vi "Main.vi"() -> ()   [LabVIEW 2017]
doc: "Use this template to build a user interface event handler design pattern. Use this pattern for dialog boxes and other user interfaces. You also can create and execute user-defined events that the VI can handle the same way as user interface events."
uses:
  <vilib>/Utility/NIReport.llb/HTML Report Image Alignment.ctl
  <vilib>/Utility/NIReport.llb/image depth.ctl
  <vilib>/addons/database/Connection.llb/DB Tools Open Connec (Path).vi
  <userlib>/_OpenG.lib/file/file.llb/File Exists - Scalar__ogtk.vi
  <vilib>/addons/database/Auxilliary.llb/DB Tools Format Datetime String (Time Stamp).vi
  GLOBAL/auto.vi
  <vilib>/Utility/NIReport.llb/Append Report Text (str wrap).vi
  <vilib>/Utility/NIReport.llb/NI_report.lvclass
  <vilib>/addons/database/NI_Database_API.lvlib
  <vilib>/Utility/NIReport.llb/NI_ReportGenerationCore.lvlib
  <vilib>/Utility/NIReport.llb/Excel/NI_Excel.lvclass
panel:
  out "columns":string[](array[string])
  in  "MAX MIN VALUES":enum32{"ACTUAL", "SET"}(tab)
  out "TEMP":cluster{"MIN":dbl, "MAX":dbl, "ACTUAL":dbl}
  out "FLOW":cluster{"MIN":dbl, "MAX":dbl, "ACTUAL":dbl}
  out "BMP":cluster{"ACTUAL":dbl}
  out "Pressure":cluster{"MIN":dbl, "MAX":dbl, "ACTUAL":dbl}
  out "TEMP SET":cluster{"MIN":dbl, "MAX":dbl, "THRESHOLD":dbl}
  out "FLOW SET":cluster{"MIN":dbl, "MAX":dbl, "THRESHOLD":dbl}
  out "BMP SET":cluster{"MIN":dbl, "MAX":dbl, "THRESHOLD":dbl}
  out "Pressure SET":cluster{"MIN":dbl, "MAX":dbl, "THRESHOLD":dbl}
  out "Loading....":u8(slide) scale=0.0..100.0
  out "BMP":bool
  out "Temp":bool
  out "Flow":bool
  out "Pressure":bool
  in  "Report":bool
  out "DESCRIPTION":string
  out "resulting string":path
  in  "import state 3":bool
  out "User Name":string
  out "Min Peak/Min":dbl
  out "Status bar":string
  in  "import state 2":bool
  out "SELECTED RECIPE":string
  out "BARCODE_FOUND":bool
  out "DB CONN":bool
  in  "Graph":bool
  out "table":string[][](table)
  out "GRAPH":cluster{timestamp[], ext[]}[](graph)
  out "TEST RESULT":bool
  in  "BARCODE":string
  out "SELECTED FILE PATH":path
  in  "Import File":bool
  in  "SELECT MEASURED FILE":i32(listbox)
  out "error out":errorcluster
  in  "File Name":string
  in  "Report Files Folder":path
  in  "Convert":bool
  in  "BROWSE FILE FOLDER":path=path "D:/ON FLOOR/Grandiose Automation/Ref Data/Test reading - 141221"
  in  "stop":bool
  # "Main"
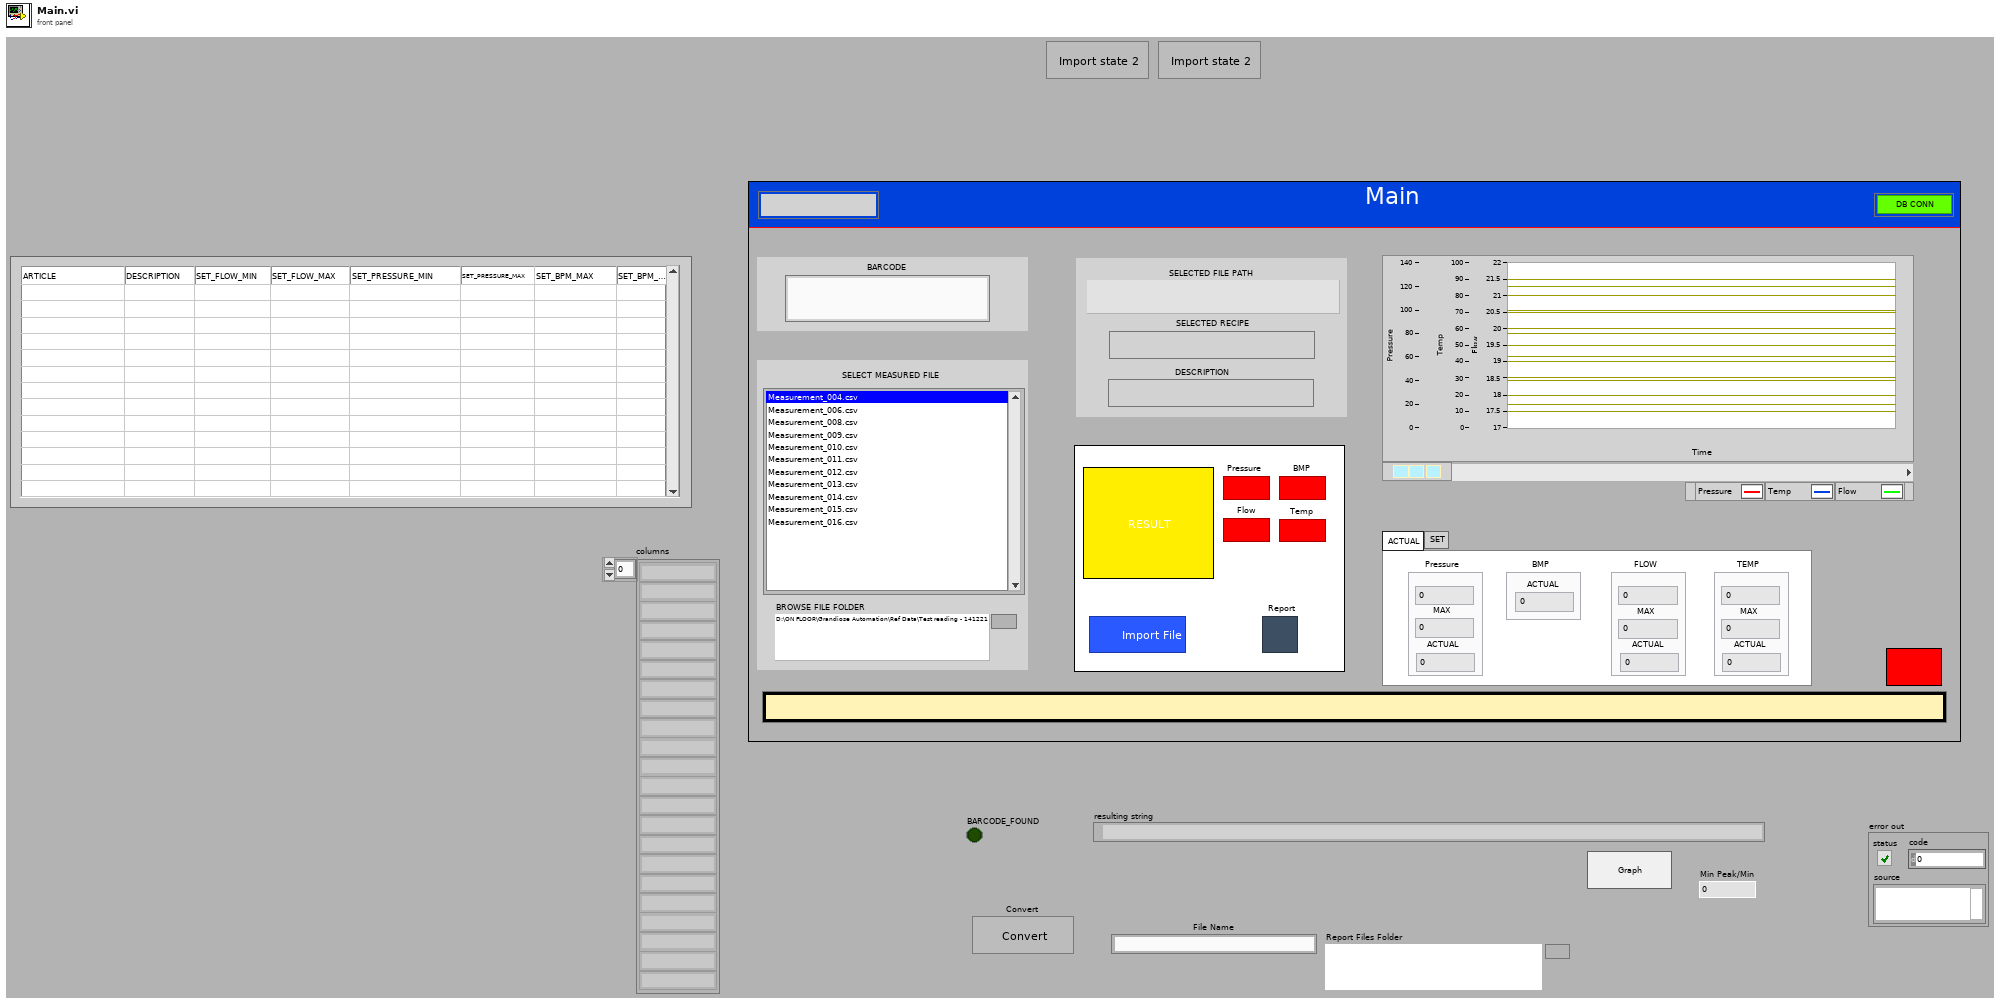
[diagram p1: front panel]
types:
  T1 = cluster{"Files":string[], "Browse File":path, "TIMEOUT":i32, "GRAPH":cluster{timestamp[], ext[]}[], "Pressure":cluster{"chl1 MIN":dbl, "chl1 MAX":dbl, "chl1 thrshold":dbl}, "Flow":cluster{"chl2 MIN":dbl, "chl2 MAX":dbl, "chl2 thrshold":dbl}, "Temp":cluster{"chl3 MIN":dbl, "chl3 MAX":dbl, "chl3 thrshold":dbl}, "Report File":path, "Data_to_report":cluster{"date/time string":string, "User Name":string, "BARCODE":string, "SELECTED RECIPE":string, "Rst":string, "Error Code":string, "RESULT ARRAY":string[]}, "BMP":cluster{"chl3 MIN":dbl, "chl3 MAX":dbl, "chl3 thrshold":dbl}}
  T2 = typedef "NI_Database_API.lvlib/Conn ObjectReference.ctl" = refnum<k1>
  T3 = enum32{"Invalid", "Standard", "Closed", "Hidden", "Minimized", "Maximized"}
  T4 = cluster{"position (Excel)":cluster{"row":i32, "column":i32}, "name (Excel)":string, "bookmark (Word)":string}[]
  T5 = cluster{"position (Excel)":cluster{"row":i32, "column":i32}, "name (Excel)":string, "bookmark (Word)":string}
  T6 = typedef "NI_ReportGenerationCore.lvlib/HTML Report Image Alignment.ctl" = enum16{"(default)", "LEFT", "RIGHT", "TOP", "TEXTTOP", "MIDDLE", "ABSMIDDLE", "BASELINE", "BOTTOM", "ABSBOTTOM"}
  T7 = enum16{"Standard Report", "HTML", "Word", "Excel"}
  T8 = enum16{"maximized", "minimized", "normal", "no change"}
  T9 = cluster{"Pressure":cluster{"chl1 MIN":dbl, "chl1 MAX":dbl, "chl1 thrshold":dbl}, "Flow":cluster{"chl2 MIN":dbl, "chl2 MAX":dbl, "chl2 thrshold":dbl}, "Temp":cluster{"chl3 MIN":dbl, "chl3 MAX":dbl, "chl3 thrshold":dbl}, "BMP":cluster{"chl3 MIN":dbl, "chl3 MAX":dbl, "chl3 thrshold":dbl}}
  T10 = cluster{"chl1 MIN":dbl, "chl1 MAX":dbl, "chl1 thrshold":dbl}
  T11 = cluster{"chl2 MIN":dbl, "chl2 MAX":dbl, "chl2 thrshold":dbl}
  T12 = cluster{"chl3 MIN":dbl, "chl3 MAX":dbl, "chl3 thrshold":dbl}
  T13 = cluster{"date/time string":string, "User Name":string, "BARCODE":string, "SELECTED RECIPE":string, "Rst":string, "Error Code 2":string}
  T14 = cluster{"date/time string":string, "User Name":string, "BARCODE":string, "SELECTED RECIPE":string, "Rst":string, "Error Code 2":string, "element":string, "element":string, "element":string, "element":string, "element":string, "element":string, "element":string, "element":string, "element":string, "element":string, "element":string}
  T15 = cluster{"date/time string":string, "User Name":string, "BARCODE":string, "SELECTED RECIPE":string, "Rst":string, "Error Code 2":string, "RESULT ARRAY":string[]}
  T16 = typedef "NI_ReportGenerationCore.lvlib/image depth.ctl" = u16
  T17 = enum32{"invalid app kind", "Development System", "Run Time System", "Student Edition", "Embedded LabVIEW", "Evaluation", "Custom"}
  T18 = cluster{"date/time string":string, "User Name":string, "BARCODE":string, "SELECTED RECIPE":string, "Rst":string, "Error Code":string, "RESULT ARRAY":string[]}
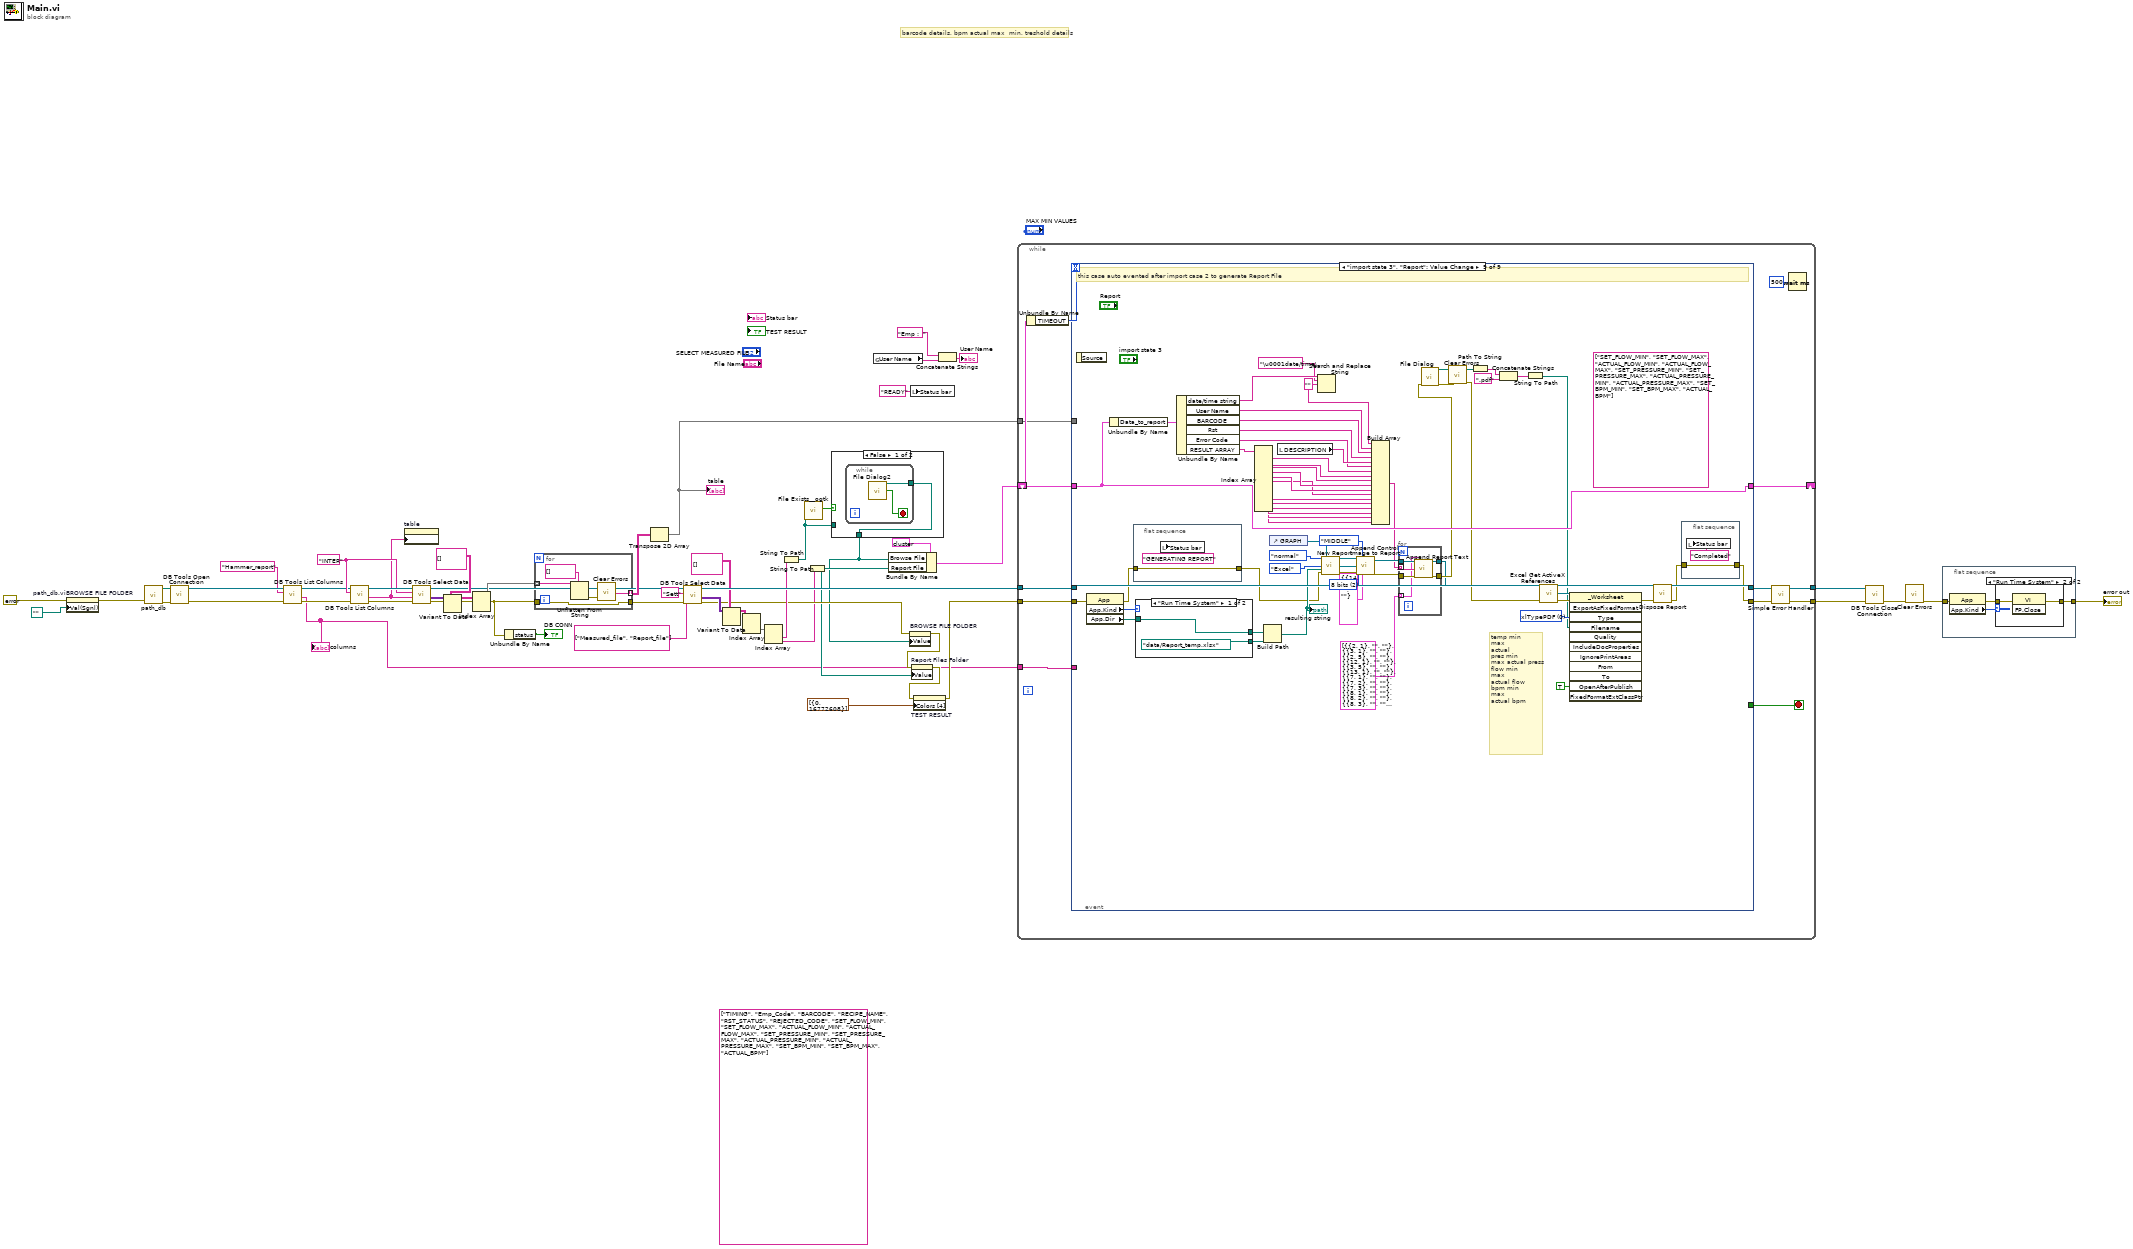
[diagram p0: block diagram]
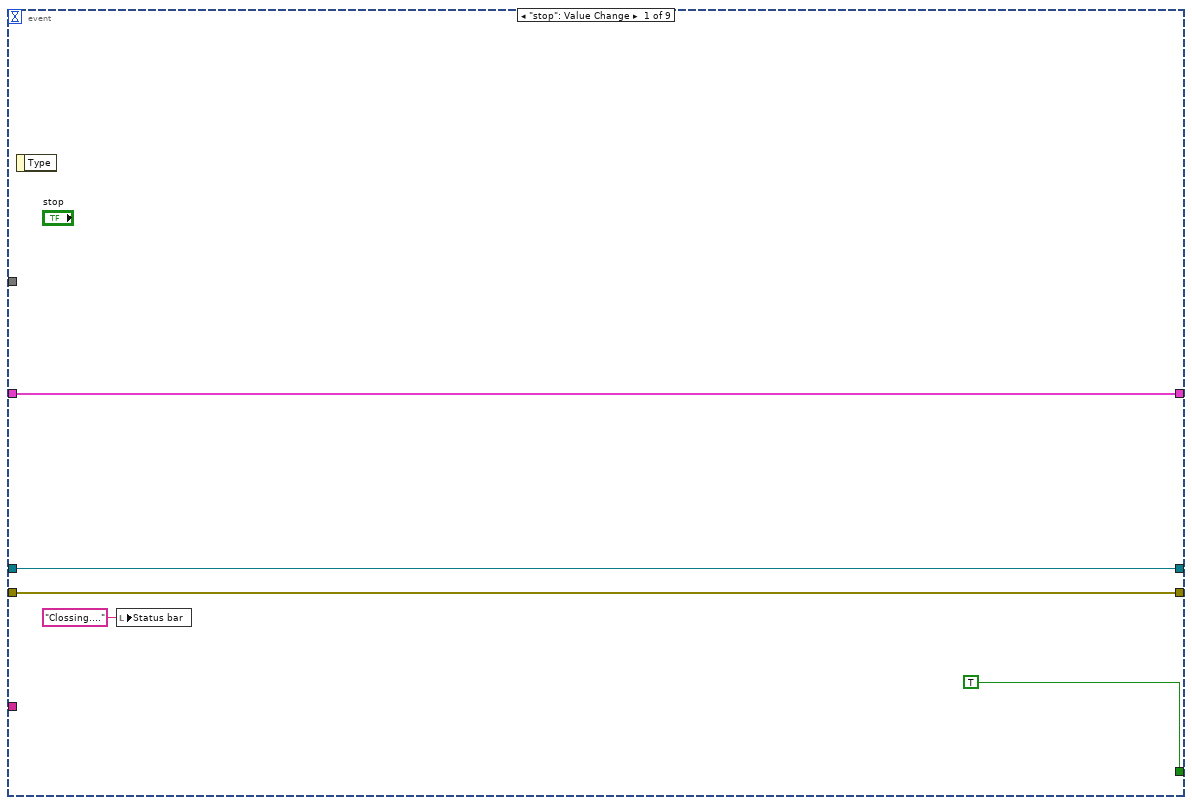
[diagram p4: hidden frame]
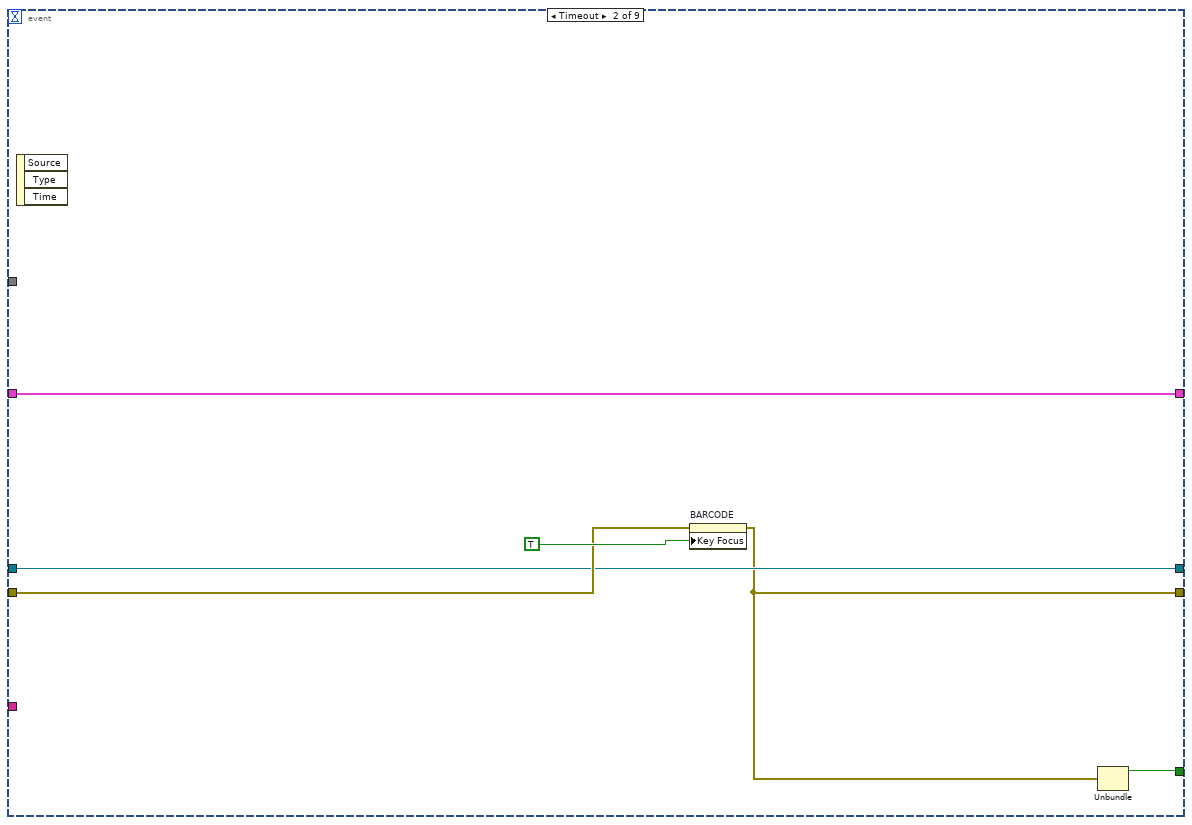
[diagram p5: hidden frame]
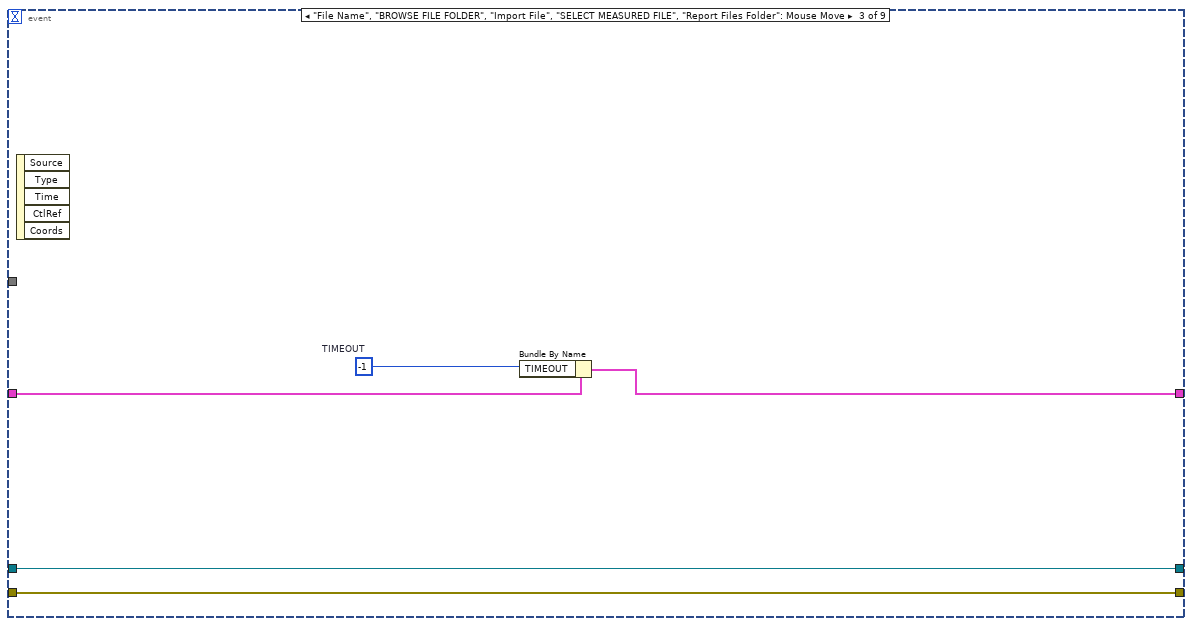
[diagram p6: hidden frame]
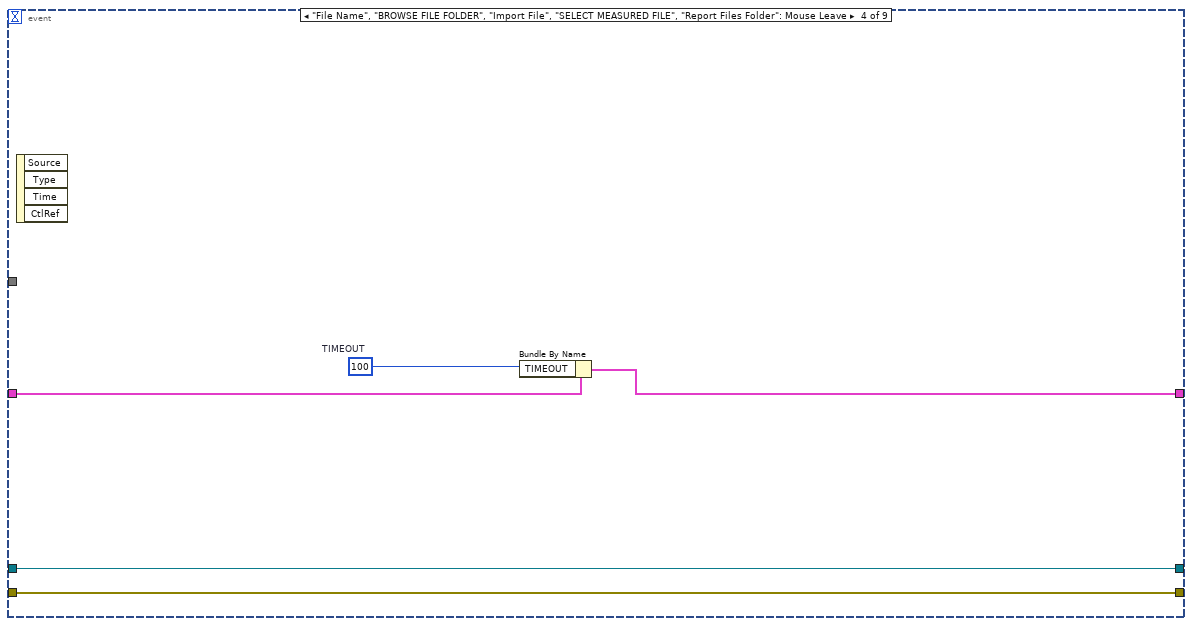
[diagram p7: hidden frame]
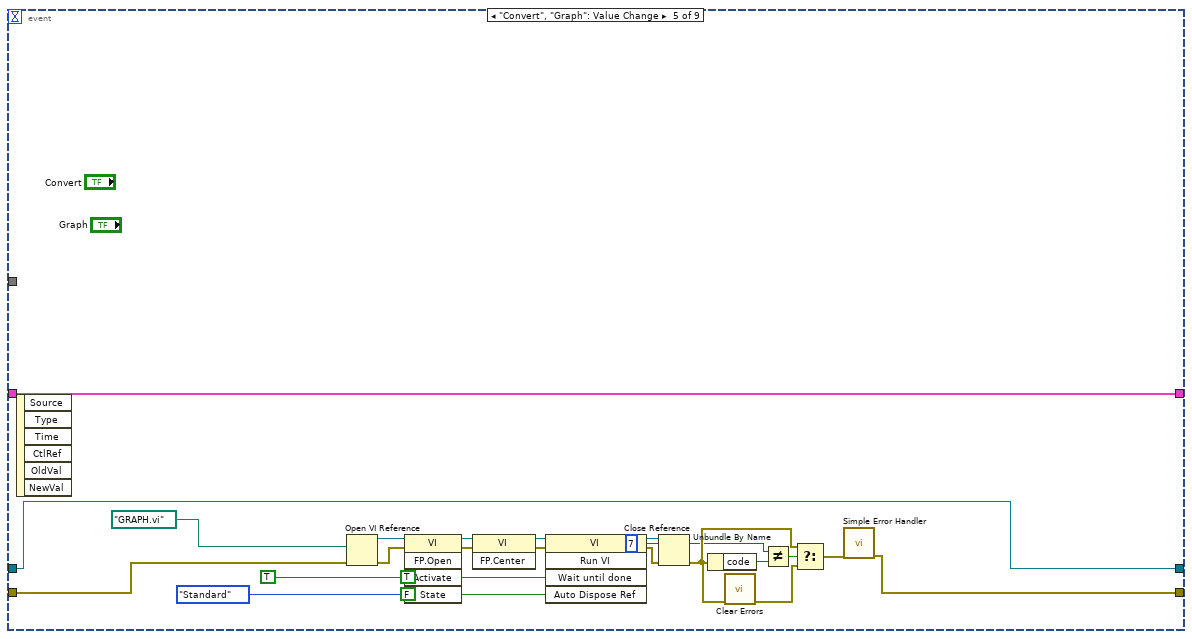
[diagram p8: hidden frame]
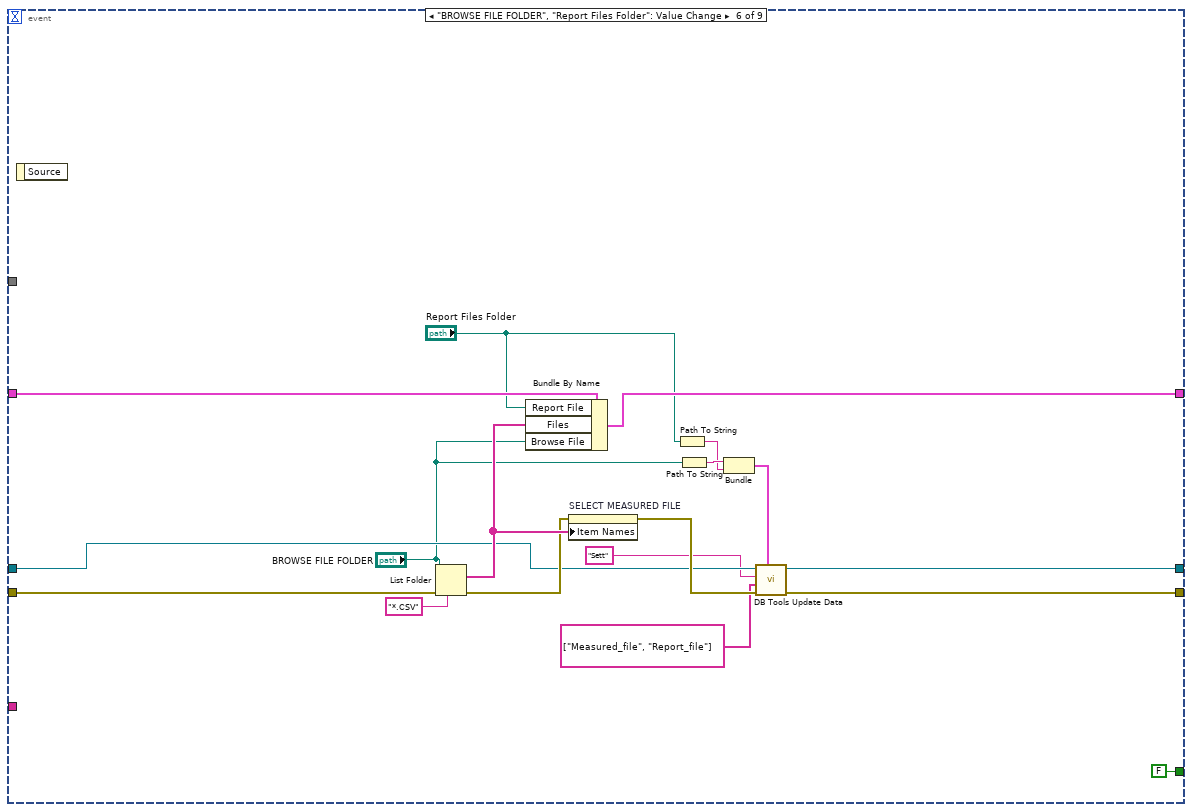
[diagram p9: hidden frame]
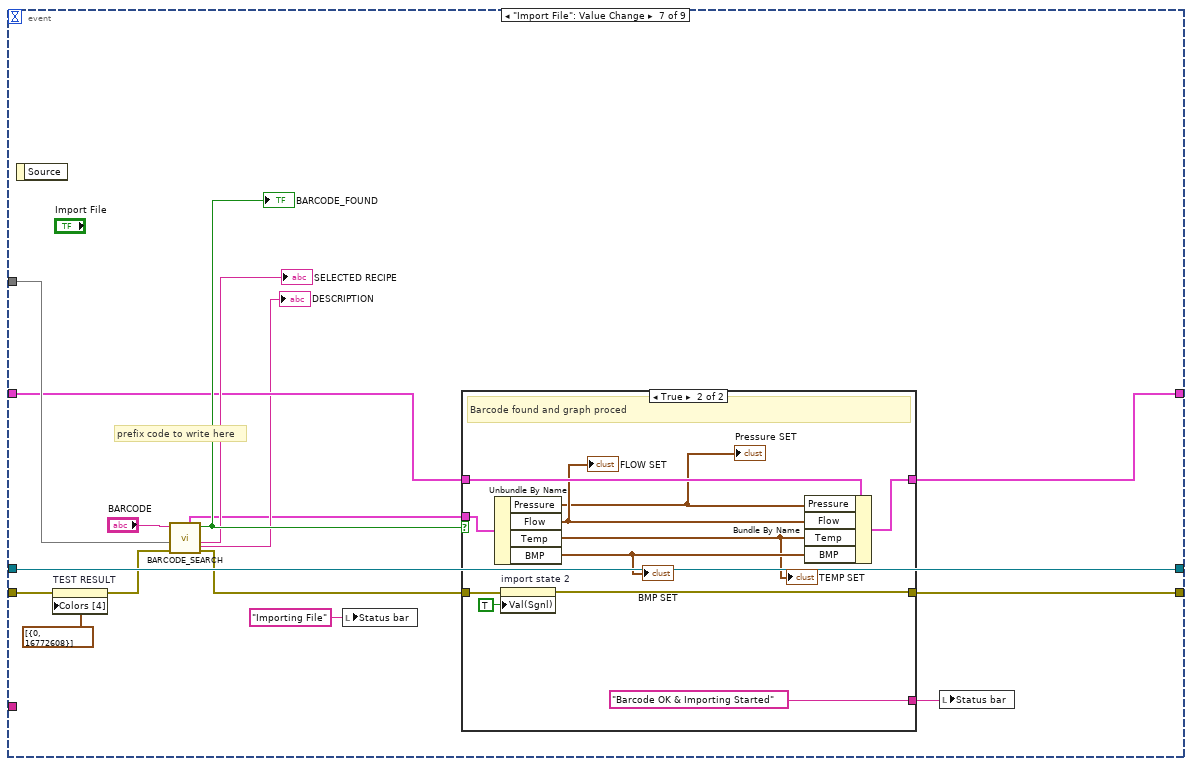
[diagram p10: hidden frame]
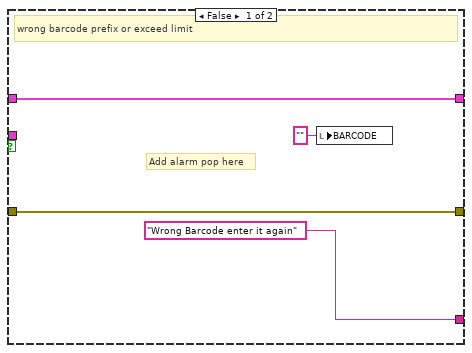
[diagram p11: hidden frame]
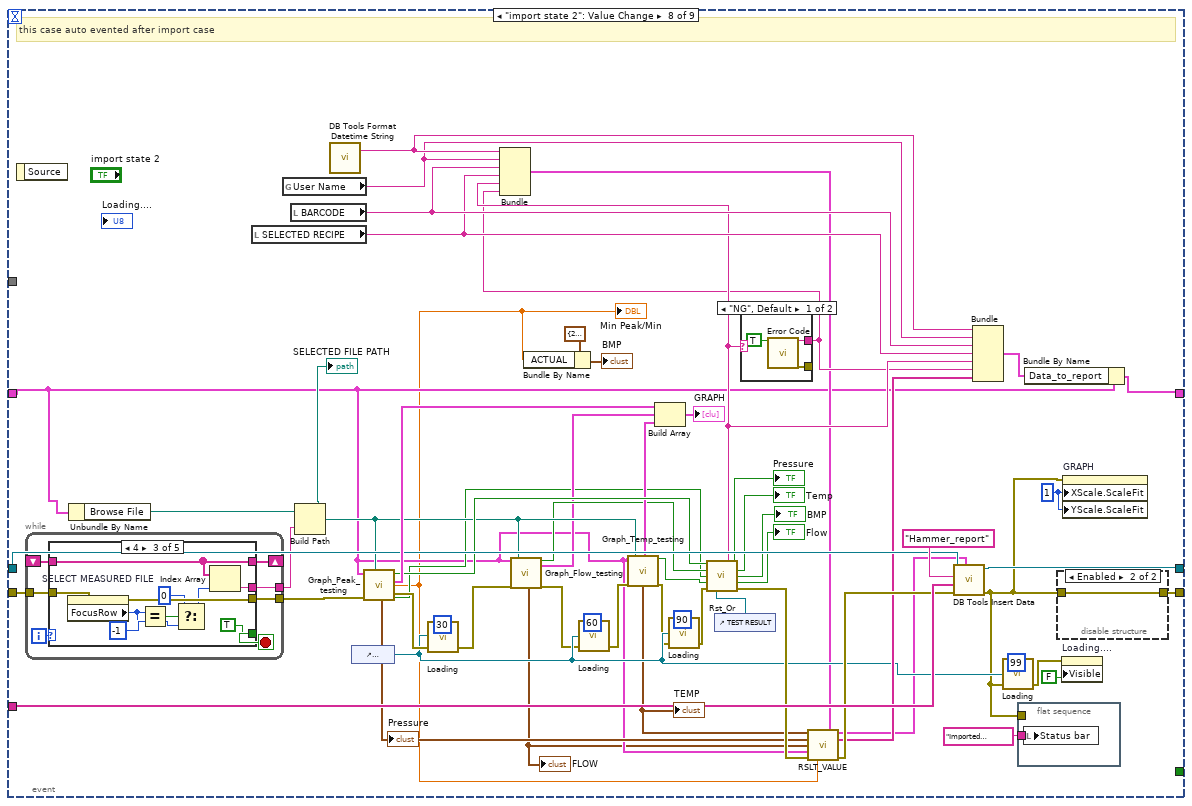
[diagram p12: hidden frame]
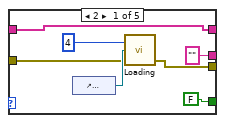
[diagram p13: hidden frame]
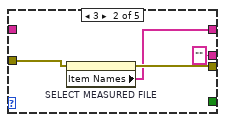
[diagram p14: hidden frame]
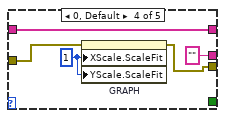
[diagram p15: hidden frame]
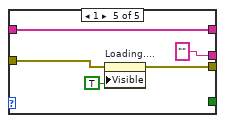
[diagram p16: hidden frame]
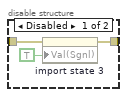
[diagram p17: hidden frame]
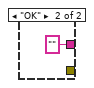
[diagram p18: hidden frame]
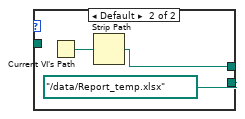
[diagram p19: hidden frame]
diagram:
  (unwired) string[] ["TIMING", "Emp_Code", "BARCODE", "RECIPE_NAME", "RST_STATUS", "REJECTED_CODE", "SET_FLOW_MIN", "SET_FLOW_MAX", "ACTUAL_FLOW_MIN", "ACTUAL_FLOW_MAX", "SET_PRESSURE_MIN", "SET_PRESSURE_MAX", "ACTUAL_PRESSURE_MIN", "ACTUAL_PRESSURE_MAX", "SET_BPM_MIN", "SET_BPM_MAX", "ACTUAL_BPM"] ("columns")
  w16 = "INTER" ("table")
  # "barcode details, bpm actual max  min, treshold details"
  n1 = property on="path_db.viBROWSE FILE FOLDER" class="Path"(error in=errorcluster {"status"=FALSE, "code"=0, "source"=""} ("error out 2"), "Val(Sgnl)"=path "" ("BROWSE FILE FOLDER")) -> (error out=w29:errorcluster)  [unwired: 1 in, 1 out]
  n2 = call "path_db.vi"("error in"=w29) -> ("error out"=w51:errorcluster, "resulting string"=w50:path)  [unwired: 9 in]
  n3 = call-poly <vilib>:"DB Tools Open Connection.vi"("error in (no error)"=w51, "connection information"=w50) -> ("error out"=w3:errorcluster, "connection reference"=w13:T2)  [unwired: 6 in]
  n4 = call <vilib>:"DB Tools List Columns.vi"("error in (no error)"=w3, "table"="Hammer_report", "connection reference"=w13) -> ("error out"=w14:errorcluster, "columns"=w10:string[], "connection reference out"=w12:T2)  [unwired: 1 in, 1 out]
  "columns" <- w10
  n5 = call <vilib>:"DB Tools List Columns.vi"("error in (no error)"=w14, "table"=w16, "connection reference"=w12) -> ("error out"=w18:errorcluster, "columns"=w7:string[], "connection reference out"=w17:T2)  [unwired: 1 in, 1 out]
  n6 = property on="table" class="Tbl (strict)"("Column Headers[]"=w7) -> ()  [unwired: 2 in, 2 out]
  n7 = call <vilib>:"DB Tools Select Data.vi"("error in (no error)"=w18, "columns"=w7, "table"=w16, "connection reference"=w17) -> ("error out"=w46:errorcluster, "data"=w53:variant[][], "connection reference out"=w41:T2)  [unwired: 2 in]
  n8 = Variant To Data(type=string[][] [], Variant=w53) -> (data=w52:string[][])  [unwired: 1 in, 1 out]
  n9 = Index Array(array=w52) -> (element=w49:string[])  [unwired: 2 in]
  n10 = Unbundle By Name(w46) -> ("status"=→"DB CONN":bool)
  n11 = for {
    tunnel: w49 -> [w58] mode=indexing
    tunnel: [w56] -> w48 mode=indexing
    tunnel: w46 -> [w55]
    tunnel: [w55] -> w42
    n12 = Unflatten From String(type=string[] [], binary string=w58) -> (value=w56:string[], error out=w59:errorcluster)  [unwired: 3 in, 1 out]
    n13 = call <vilib>:"Clear Errors.vi"("error in (no error)"=w59) -> ()  [unwired: 5 in, 2 out]
  }
  n14 = Transpose 2D Array(2D array=w48) -> (transposed array=w27:string[][])
  "table" <- w27
  n15 = call <vilib>:"DB Tools Select Data.vi"("error in (no error)"=w42, "columns"=string[] ["Measured_file", "Report_file"], "table"="Sett", "connection reference"=w41) -> ("error out"=w31:errorcluster, "data"=w39:variant[][], "connection reference out"=w40:T2)  [unwired: 2 in]
  n16 = Variant To Data(type=string[][] [], Variant=w39) -> (data=w37:string[][])  [unwired: 1 in, 1 out]
  n17 = Index Array(array=w37) -> (element=w33:string[])  [unwired: 2 in]
  n18 = Index Array(array=w33) -> (element #1=w32:string, element #2=w26:string)  [unwired: 2 in]
  n19 = String To Path(string=w32) -> (path=w5:path)
  n20 = call-poly <userlib>:"File Exists__ogtk.vi"("file path"=w5) -> ("is directory"=w6:bool)  [unwired: 6 in, 1 out]
  n21 = String To Path(string=w26) -> (path=w25:path)
  n22 = case shown="False" w6 {
    tunnel: [w60 w63] -> w4
    tunnel: w5 -> [_ w63]
    frame False {
      n23 = while {
        tunnel: [w61] -> w60
        stop <- w62 stop-if-true
        n24 = call "File Dialog2"() -> ("selected path"=w61:path, "exists"=w62:bool)  [unwired: 12 in, 2 out]
      }
    }
    frame True {
    }
  }
  n25 = global read "auto.vi" "User Name"() -> (w9:string)
  n26 = Bundle By Name(cluster=T1 {"Files"=[], "Browse File"=path "", "TIMEOUT"=100, "GRAPH"=[{array[68443 elements], array[68443 elements]}, {array[68363 elements], array[68363 elements]}, {array[40500 elements], array[40500 elements]}], "Pressure"={"chl1 MIN"=110.0, "chl1 MAX"=130.0, "chl1 thrshold"=120.0}, "Flow"={"chl2 MIN"=33.0, "chl2 MAX"=35.0, "chl2 thrshold"=25.0}, "Temp"={"chl3 MIN"=20.0, "chl3 MAX"=30.0, "chl3 thrshold"=34.0}, "Report File"=path "", "Data_to_report"={"date/time string"="", "User Name"="", "BARCODE"="", "SELECTED RECIPE"="", "Rst"="", "Error Code"="", "RESULT ARRAY"=[]}, "BMP"={"chl3 MIN"=1000.0, "chl3 MAX"=2000.0, "chl3 thrshold"=0.0}}, "Browse File"=w4, "Report File"=w25) -> (w34:T1)
  n27 = property on="BROWSE FILE FOLDER" class="Path"(error in=w31, "Value"=w4) -> (error out=w24:errorcluster)  [unwired: 1 in, 1 out]
  n28 = local write "Status bar"("READY" ("Status bar")) -> ()
  n29 = property on="Report Files Folder" class="Path"(error in=w24, "Value"=w25) -> (error out=w23:errorcluster)  [unwired: 1 in, 1 out]
  n30 = property on="TEST RESULT" class="Bool"(error in=w23, "Colors [4]"=cluster{u32, u32}[] [{0, 16772608}]) -> (error out=w20:errorcluster)  [unwired: 1 in, 1 out]
  n31 = Concatenate Strings("Emp :  " ("string"), w9) -> (→"User Name":string)
  n32 = while {
    tunnel: w20 -> [w73]
    tunnel: [w65] -> w45
    shift-right: [w72] -> _
    shift-left: w34 -> [w70]
    tunnel: w40 -> [w68]
    tunnel: [w69] -> w44
    tunnel: w27 -> [w67]
    tunnel: w10 -> [w64]
    stop <- w75 stop-if-true
    n33 = Unbundle By Name(w70) -> ("TIMEOUT"=w71:i32)
    n34 = event shown="[8] \"import state 3\", \"Report\": Value Change" {
      selector: _ -> [_ _ _ _ _ _ _ _ _]
      dyn-events: _ -> [_ _ _ _ _ _ _ _ _]
      timeout: w71 -> [_ _ _ _ _ _ _ _ _]
      tunnel: [TRUE w81 _ _ _ FALSE _ _ _] -> w75
      tunnel: w73 -> [w79 w84 w91 w96 w99 w137 w143 w204 w331]
      tunnel: [w79 w82 w91 w96 w98 w130 w150 w221 w316] -> w66
      tunnel: w70 -> [w80 w86 w90 w95 w119 w136 w146 w175 w321]
      tunnel: [w80 w86 w89 w94 w119 w135 w145 w220 w321] -> w72
      tunnel: [w77 w83 w87 w92 w97 w128 w153 w222 w336] -> w69
      tunnel: w68 -> [w77 w83 w87 w92 w97 w129 w153 w223 w336]
      tunnel: w67 -> [_ _ _ _ _ _ w147 _ _]
      tunnel: w64 -> [_ _ _ _ _ _ _ w218 _]
      event "stop": Value Change {
        n35 = event-data() -> ()  [unwired: 1 in, 1 out]
        n36 = local write "Status bar"("Clossing...." ("Status bar")) -> ()
      }
      event Timeout {
        n37 = event-data() -> ()  [unwired: 1 in, 3 out]
        n38 = property on="BARCODE" class="Str"(error in=w84, "Key Focus"=TRUE) -> (error out=w82:errorcluster)  [unwired: 1 in, 1 out]
        n39 = Unbundle(w82) -> ("status"=w81:bool)  [unwired: 2 out]
      }
      event "File Name", "BROWSE FILE FOLDER", "Import File", "SELECT MEASURED FILE", "Report Files Folder": Mouse Move {
        w88 = -1  # TIMEOUT
        n40 = event-data() -> ()  [unwired: 1 in, 5 out]
        n41 = Bundle By Name(cluster=w90, "TIMEOUT"=w88) -> (w89:T1)
      }
      event "File Name", "BROWSE FILE FOLDER", "Import File", "SELECT MEASURED FILE", "Report Files Folder": Mouse Leave {
        w93 = 100  # TIMEOUT
        n42 = event-data() -> ()  [unwired: 1 in, 4 out]
        n43 = Bundle By Name(cluster=w95, "TIMEOUT"=w93) -> (w94:T1)
      }
      event "Convert", "Graph": Value Change {
        n44 = event-data() -> ()  [unwired: 1 in, 6 out]
        n45 = Open VI Reference(vi path=path "GRAPH.vi", error in (no error)=w99) -> (vi reference=w106:refnum<vi>, error out=w118:errorcluster)  [unwired: 4 in]
        n46 = invoke class="VI" method="FP.Open"(reference=w106, error in=w118, "Activate"=TRUE ("Activate?"), "State"=T3."Standard") -> (reference out=w117:refnum<vi>, error out=w112:errorcluster)  [unwired: 1 in, 3 out]
        n47 = invoke class="VI" method="FP.Center"(reference=w117, error in=w112) -> (reference out=w113:refnum<vi>, error out=w114:errorcluster)  [unwired: 1 in, 1 out]
        n48 = invoke class="VI" method="Run VI"(reference=w113, error in=w114, "Wait until done"=TRUE ("Wait Until Done"), "Auto Dispose Ref"=FALSE ("Auto Dispose Reference")) -> (reference out=w115:refnum<vi>, error out=w116:errorcluster)  [unwired: 1 in, 3 out]
        n49 = Close Reference(reference=w115, error in (no error)=w116) -> (error out=w107:errorcluster)
        n50 = Unbundle By Name(w107) -> ("code"=w111:i32)
        n51 = call <vilib>:"Clear Errors.vi"("error in (no error)"=w107) -> ("error out"=w109:errorcluster)  [unwired: 5 in, 1 out]
        n52 = Not Equal?(x=7, y=w111) -> (x != y?=w110:bool)
        n53 = Select(t=w107, s=w110, f=w109) -> (s? t:f=w108:errorcluster)
        n54 = call <vilib>:"Simple Error Handler.vi"("error in (no error)"=w108) -> ("error out"=w98:errorcluster)  [unwired: 4 in, 4 out]
      }
      event "BROWSE FILE FOLDER", "Report Files Folder": Value Change {
        n55 = event-data() -> ()  [unwired: 1 in, 1 out]
        n56 = List Folder(path="BROWSE FILE FOLDER", pattern="*.CSV", error in=w137) -> (filenames=w133:string[], error out=w132:errorcluster)  [unwired: 1 in, 2 out]
        n57 = Bundle By Name(cluster=w136, "Report File"="Report Files Folder", "Files"=w133, "Browse File"="BROWSE FILE FOLDER") -> (w135:T1)
        n58 = property on="SELECT MEASURED FILE" class="LstBox (strict)"(error in=w132, "Item Names"=w133) -> (error out=w131:errorcluster)  [unwired: 1 in, 1 out]
        n59 = Path To String(path="Report Files Folder") -> (string=w122:string)
        n60 = Path To String(path="BROWSE FILE FOLDER") -> (string=w124:string)
        n61 = Bundle(w124, w122) -> (w127:cluster{string, string})  [unwired: 1 in]
        n62 = call <vilib>:"DB Tools Update Data.vi"("data"=w127, "error in (no error)"=w131, "columns"=string[] ["Measured_file", "Report_file"], "table"="Sett", "connection reference"=w129) -> ("error out"=w130:errorcluster, "connection reference out"=w128:T2)  [unwired: 5 in]
      }
      event "Import File": Value Change {
        # "prefix code to write here"
        n63 = event-data() -> ()  [unwired: 1 in, 1 out]
        n64 = property on="TEST RESULT" class="Bool"(error in=w143, "Colors [4]"=cluster{u32, u32}[] [{0, 16772608}]) -> (error out=w142:errorcluster)  [unwired: 1 in, 1 out]
        n65 = call "BARCODE_SEARCH.vi"("error in"=w142, "BARCODE_TABLE"=w147, "BARCODE_TO_SEARCH"="BARCODE") -> ("error out"=w151:errorcluster, "ARTICLE name"=→"SELECTED RECIPE":string, "BARCODE_FOUND"=w149:bool, "description NAME"=→"DESCRIPTION":string, "CHL"=w138:T9)  [unwired: 3 in, 1 out]
        "BARCODE_FOUND" <- w149
        n66 = local write "Status bar"("Importing File" ("Status bar")) -> ()
        n67 = case shown="True" w149 {
          tunnel: [w157 w166] -> w150
          tunnel: w151 -> [w157 w167]
          tunnel: [w156 w164] -> w145
          tunnel: w146 -> [w156 w165]
          tunnel: ["Wrong Barcode enter it again" ("Status bar") "Barcode OK & Importing Started" ("Status bar")] -> w140
          tunnel: w138 -> [_ w162]
          frame False {
            # "Add alarm pop here"
            # "wrong barcode prefix or exceed limit"
            n68 = local write "BARCODE"("" ("BARCODE")) -> ()
          }
          frame True {
            # "Barcode found and graph proced"
            n69 = Unbundle By Name(w162) -> ("Pressure"=w158:T10, "Flow"=w159:T11, "Temp"=w160:T12, "BMP"=w161:T12)
            "Pressure SET" <- w158
            "BMP SET" <- w161
            "FLOW SET" <- w159
            "TEMP SET" <- w160
            n70 = property on="import state 2" class="Bool (strict)"(error in=w167, "Val(Sgnl)"=TRUE) -> (error out=w166:errorcluster)  [unwired: 1 in, 1 out]
            n71 = Bundle By Name(cluster=w165, "Pressure"=w158, "Flow"=w159, "Temp"=w160, "BMP"=w161) -> (w164:T1)
          }
        }
        n72 = local write "Status bar"(w140) -> ()
      }
      event "import state 2": Value Change {
        w171 = u8 1 ("X Scale.Scale Fit")
        # "this case auto evented after import case"
        n73 = event-data() -> ()  [unwired: 1 in, 1 out]
        n74 = while {
          tunnel: [w234] -> w203
          tunnel: w204 -> [w233]
          shift-right: [w230] -> _
          shift-left: _ -> [w229]
          tunnel: [w228] -> w202
          i -> [w232]
          stop <- w231 stop-if-true
          n75 = case shown="4" w232 {
            tunnel: [w239 w245 w254 w257 w264] -> w234
            tunnel: w233 -> [w238 w244 w255 w256 w263]
            tunnel: [FALSE _ TRUE _ _] -> w231
            tunnel: [w236 w243 w248 w259 w262] -> w230
            tunnel: w229 -> [w236 _ w248 w259 w262]
            tunnel: ["" "" w247 "" ""] -> w228
            frame 2 {
              n76 = control-ref of="Loading...."() -> (w241:refnum<vi>)
              n77 = call "Loading.vi"("error in"=w238, "reference"=w241, "Value"=u8 4) -> ("error out"=w239:errorcluster)  [unwired: 2 in]
            }
            frame 3 {
              n78 = property on="SELECT MEASURED FILE" class="LstBox (strict)"(error in=w244) -> (error out=w245:errorcluster, "Item Names"=w243:string[])  [unwired: 1 in, 1 out]
            }
            frame 4 {
              n79 = property on="SELECT MEASURED FILE" class="LstBox (strict)"(error in=w255) -> (error out=w254:errorcluster, "FocusRow"=w250:i32)  [unwired: 1 in, 1 out]
              n80 = Equal?(x=w250, y=-1) -> (x = y?=w253:bool)
              n81 = Select(t=0 ("y"), s=w253, f=w250) -> (s? t:f=w249:i32)
              n82 = Index Array(array=w248, index=w249) -> (element=w247:string)
            }
            frame 0, Default {
              w260 = u8 1 ("X Scale.Scale Fit")
              n83 = property on="GRAPH" class="XYGraph (strict)"(error in=w256, "XScale.ScaleFit"=w260, "YScale.ScaleFit"=w260) -> (error out=w257:errorcluster)  [unwired: 1 in, 1 out]
            }
            frame 1 {
              n84 = property on="Loading...." class="Slide (strict)"(error in=w263, "Visible"=TRUE) -> (error out=w264:errorcluster)  [unwired: 1 in, 1 out]
            }
          }
        }
        n85 = Unbundle By Name(w175) -> ("Browse File"=w227:path)
        n86 = local read "SELECTED RECIPE"() -> (w181:string)
        n87 = global read "auto.vi" "User Name"() -> (w183:string)
        n88 = local read "BARCODE"() -> (w182:string)
        n89 = Build Path(base path=w227, name or relative path=w202) -> (appended path=w197:path)
        "SELECTED FILE PATH" <- w197
        n90 = call-poly <vilib>:"DB Tools Format Datetime String.vi"() -> ("date/time string"=w184:string)  [unwired: 1 in]
        n91 = control-ref of="Loading...."() -> (w207:refnum<vi>)
        n92 = call "Graph_Peak_testing.vi"("CSV file path"=w197, "error in"=w203, "Cluster"=w175) -> ("MIN_MAX_BPM"=w186:bool, "Filter Graph"=w225:cluster{timestamp[], ext[]}, "MIN_MAX_PRESSURE"=w205:bool, "ACTUAL BPM"=w169:dbl, "error out"=w211:errorcluster, "MAX_MIN_PRESSURE"=w189:cluster{"MIN":dbl, "MAX":dbl, "ACTUAL":dbl})  [unwired: 1 in, 1 out]
        "Min Peak/Min" <- w169
        "Pressure" <- w189
        n93 = call "Loading.vi"("error in"=w211, "reference"=w207, "Value"=u8 30) -> ("error out"=w195:errorcluster)  [unwired: 2 in]
        n94 = call "Graph_Flow_testing.vi"("Cluster"=w175, "error in"=w195, "CSV file path"=w197) -> ("MIN_MAX_FLOW"=w196:bool, "Filter Graph Flow"=w193:cluster{timestamp[], ext[]}, "MAX-MIN_Flow"=w174:cluster{"MIN":dbl, "MAX":dbl, "ACTUAL":dbl}, "error out"=w194:errorcluster)  [unwired: 13 in]
        "FLOW" <- w174
        n95 = Bundle By Name(cluster=cluster{"ACTUAL":dbl} {"ACTUAL"=21.503} ("BMP 2"), "ACTUAL"=w169) -> (→"BMP":cluster{"ACTUAL":dbl})
        n96 = call "Loading.vi"("error in"=w194, "reference"=w207, "Value"=u8 60) -> ("error out"=w201:errorcluster)  [unwired: 2 in]
        n97 = call "Graph_Temp_testing.vi"("Cluster"=w175, "error in"=w201, "CSV file path"=w197) -> (14:"MAX-MIN_Temp"=w199:bool, "Filter Graph"=w200:cluster{timestamp[], ext[]}, 16:"MAX-MIN_Temp"=w173:cluster{"MIN":dbl, "MAX":dbl, "ACTUAL":dbl}, "error out"=w198:errorcluster)  [unwired: 13 in]
        "TEMP" <- w173
        n98 = Build Array(w225, w193, w200) -> (→"GRAPH":cluster{timestamp[], ext[]}[])
        n99 = call "Loading.vi"("error in"=w198, "reference"=w207, "Value"=u8 90) -> ("error out"=w210:errorcluster)  [unwired: 2 in]
        n100 = control-ref of="TEST RESULT"() -> (w176:refnum<vi>)
        n101 = call "Rst_Or.vi"("BAR rst"=w205, "L/Min rst"=w196, "BPM rst"=w186, "A*C rst"=w199, "error In"=w210, "RST_COLOR"=w176) -> ("Rst"=w180:string, "BAR"=→"Pressure":bool, "L/Min"=→"Temp":bool, "BPM"=→"BMP":bool, "A*C"=→"Flow":bool, "error out"=w217:errorcluster)  [unwired: 4 in]
        n102 = case shown="\"NG\", Default" w180 {
          tunnel: [w273 ""] -> w179
          tunnel: [w272 _] -> _
          frame "NG", Default {
            n103 = call "Error Code.vi"("Enable"=TRUE) -> ("Error Code 2"=w273:string, "error out"=w272:errorcluster)  [unwired: 16 in, 1 out]
          }
          frame "OK" {
          }
        }
        n104 = Bundle("date/time string"=w184, "User Name"=w183, "BARCODE"=w182, "SELECTED RECIPE"=w181, "Rst"=w180, "Error Code 2"=w179) -> (w178:T13)  [unwired: 1 in]
        n105 = call "RSLT_VALUE.vi"("MAX-MIN Temp"=w173, "INPUT cluster"=w178, "MAX-MIN PRESSURE"=w189, "MAX-MIN FLOW"=w174, "CLUSTER"=w175, "error in"=w217, "ACTUAL BPM"=w169) -> ("CLUSTER TO SQL"=w177:T14, "RESULT ARRAY"=w215:string[], "error OUT"=w216:errorcluster)  [unwired: 6 in]
        n106 = call <vilib>:"DB Tools Insert Data.vi"("data"=w177, "error in (no error)"=w216, "columns"=w218, "table"="Hammer_report", "connection reference"=w223) -> ("error out"=w170:errorcluster, "connection reference out"=w222:T2)  [unwired: 5 in]
        n107 = Bundle("date/time string"=w184, "User Name"=w183, "BARCODE"=w182, "SELECTED RECIPE"=w181, "Rst"=w180, "Error Code 2"=w179, "RESULT ARRAY"=w215) -> (w214:T15)  [unwired: 1 in]
        n108 = call "Loading.vi"("error in"=w170, "reference"=w207, "Value"=u8 99) -> ("error out"=w172:errorcluster)  [unwired: 2 in]
        n109 = flat-sequence {
          tunnel: "Imported Completed & Click on Generate Report button for Report" ("Status bar") -> [w266]
          tunnel: w170 -> [_]
          frame #0 {
            n110 = local write "Status bar"(w266) -> ()
          }
        }
        n111 = Bundle By Name(cluster=w175, "Data_to_report"=w214) -> (w220:T1)
        n112 = disable-structure shown="Enabled" {
          disable-tunnel: w170 -> [w269 w270]
          disable-tunnel: [w268 w270] -> w221
          frame Disabled {
            n113 = property on="import state 3" class="Bool (strict)"(error in=w269, "Val(Sgnl)"=TRUE) -> (error out=w268:errorcluster)  [unwired: 1 in, 1 out]
          }
          frame Enabled {
          }
        }
        n114 = property on="Loading...." class="Slide (strict)"(error in=w172, "Visible"=FALSE) -> ()  [unwired: 1 in, 2 out]
        n115 = property on="GRAPH" class="XYGraph (strict)"(error in=w170, "XScale.ScaleFit"=w171, "YScale.ScaleFit"=w171) -> ()  [unwired: 1 in, 2 out]
      }
      event "import state 3", "Report": Value Change {
        w283 = 0 items=["xlTypePDF", "xlTypeXPS"] ("Type")
        (unwired) string[] ["SET_FLOW_MIN", "SET_FLOW_MAX", "ACTUAL_FLOW_MIN", "ACTUAL_FLOW_MAX", "SET_PRESSURE_MIN", "SET_PRESSURE_MAX", "ACTUAL_PRESSURE_MIN", "ACTUAL_PRESSURE_MAX", "SET_BPM_MIN", "SET_BPM_MAX", "ACTUAL_BPM"] ("columns")
        w322 = T16 2 items=["B&W", "4 bits", "8 bits", "24 bits"] ("image depth")
        # "temp min\nmax\nactual\npres min\nmax actual press\nflow min\nmax\nactual flow\nbpm min\nmax\nactual bpm"
        # "this case auto evented after import case 2 to generate Report File"
        n116 = event-data() -> ()  [unwired: 1 in, 1 out]
        n117 = property class="App"(error in=w331) -> (error out=w318:errorcluster, "App.Kind"=w335:T17, "App.Dir"=w334:path)  [unwired: 1 in, 1 out]
        n118 = Unbundle By Name(w321) -> ("Data_to_report"=w304:T18)
        n119 = flat-sequence {
          tunnel: w318 -> [w345]
          tunnel: [w345] -> w317
          frame #0 {
            n120 = local write "Status bar"("GENERATING REPORT" ("Status bar")) -> ()
          }
        }
        n121 = case shown="\"Run Time System\"" w335 {
          tunnel: w334 -> [w348 _]
          tunnel: [path "data/Report_temp.xlsx" ("path") path "../data/Report_temp.xlsx" ("path")] -> w333
          tunnel: [w348 w349] -> w332
          frame "Run Time System" {
          }
          frame Default {
            n122 = Current VI's Path() -> (path=w350:path)
            n123 = Strip Path(path=w350) -> (stripped path=w349:path)  [unwired: 1 out]
          }
        }
        n124 = Unbundle By Name(w304) -> ("date/time string"=w288:string, "User Name"=w305:string, "BARCODE"=w306:string, "Rst"=w307:string, "Error Code"=w302:string, "RESULT ARRAY"=w301:string[])
        n125 = Index Array(array=w301) -> (element #1=w300:string, element #2=w299:string, element #3=w298:string, element #4=w297:string, element #5=w296:string, element #6=w295:string, element #7=w294:string, element #8=w293:string, element #9=w292:string, element #10=w291:string, element #11=w290:string, element #12=w289:string)  [unwired: 12 in]
        n126 = Build Path(base path=w332, name or relative path=w333) -> (appended path=w327:path)
        "resulting string" <- w327
        n127 = control-ref of="GRAPH"() -> (w330:refnum<vi>)
        n128 = local read "DESCRIPTION"() -> (w303:string)
        n129 = Search and Replace String(input string=w288, search string="\u0001date/time\u0001", replace string="" ("replace string (\"\")")) -> (result string=w285:string)  [unwired: 5 in, 3 out]
        n130 = call <vilib>:"New Report.vi"("window state (normal)"=T8."normal", "report type"=T7."Excel", "template (empty)"=w327, "error in (no error)"=w317) -> ("report out"=w329:refnum<class "NI_report.lvclass">, "error out"=w328:errorcluster)  [unwired: 10 in]
        n131 = call-dynamic "Append Control Image to Report.vi"("report in"=w329, "alignment (default)"=HTML_Report_Image_Alignment."MIDDLE", "image depth"=w322, "ctrl reference"=w330, "error in (no error)"=w328, "MS Office parameters"=T5 {"position (Excel)"={"row"=14, "column"=0}, "name (Excel)"="", "bookmark (Word)"=""}) -> ("report out"=w320:refnum<class "NI_report.lvclass">, "error out"=w319:errorcluster)  [unwired: 6 in, 2 out]
        n132 = Build Array(w285, w305, w306, w307, w303, w302, w300, w299, w298, w297, w296, w295, w294, w293, w292, w291, w290, w289) -> (w308:string[])
        n133 = for {
          tunnel: w308 -> [w340] mode=indexing
          tunnel: T4 [{"position (Excel)"={"row"=2, "column"=1}, "name (Excel)"="", "bookmark (Word)"=""}, {"position (Excel)"={"row"=3, "column"=1}, "name (Excel)"="", "bookmark (Word)"=""}, {"position (Excel)"={"row"=2, "column"=5}, "name (Excel)"="", "bookmark (Word)"=""}, {"position (Excel)"={"row"=12, "column"=1}, "name (Excel)"="", "bookmark (Word)"=""}, {"position (Excel)"={"row"=3, "column"=5}, "name (Excel)"="", "bookmark (Word)"=""}, {"position (Excel)"={"row"=13, "column"=1}, "name (Excel)"="", "bookmark (Word)"=""}, {"position (Excel)"={"row"=7, "column"=1}, "name (Excel)"="", "bookmark (Word)"=""}, {"position (Excel)"={"row"=7, "column"=2}, "name (Excel)"="", "bookmark (Word)"=""}, {"position (Excel)"={"row"=7, "column"=3}, "name (Excel)"="", "bookmark (Word)"=""}, {"position (Excel)"={"row"=8, "column"=1}, "name (Excel)"="", "bookmark (Word)"=""}, {"position (Excel)"={"row"=8, "column"=2}, "name (Excel)"="", "bookmark (Word)"=""}, {"position (Excel)"={"row"=8, "column"=3}, "name (Excel)"="", "bookmark (Word)"=""}, {"position (Excel)"={"row"=9, "column"=1}, "name (Excel)"="", "bookmark (Word)"=""}, {"position (Excel)"={"row"=9, "column"=2}, "name (Excel)"="", "bookmark (Word)"=""}, {"position (Excel)"={"row"=9, "column"=3}, "name (Excel)"="", "bookmark (Word)"=""}, {"position (Excel)"={"row"=10, "column"=1}, "name (Excel)"="", "bookmark (Word)"=""}, {"position (Excel)"={"row"=10, "column"=2}, "name (Excel)"="", "bookmark (Word)"=""}, {"position (Excel)"={"row"=10, "column"=3}, "name (Excel)"="", "bookmark (Word)"=""}] ("MS Office parameters") -> [w337] mode=indexing
          tunnel: w320 -> [w341]
          tunnel: [w339] -> w277
          tunnel: w319 -> [w342]
          tunnel: [w338] -> w280
          n134 = call-poly <vilib>:"Append Report Text.vi"("report in"=w341, "MS Office parameters"=w337, "text"=w340, "error in (no error)"=w342) -> ("report out"=w339:refnum<class "NI_report.lvclass">, "error out"=w338:errorcluster)  [unwired: 8 in, 2 out]
        }
        n135 = call "File Dialog"("error in"=w280) -> ("selected path"=w314:path, "error out"=w310:errorcluster)  [unwired: 11 in, 2 out]
        n136 = call <vilib>:"Clear Errors.vi"("error in (no error)"=w310) -> ("error out"=w279:errorcluster)  [unwired: 5 in, 1 out]
        n137 = Path To String(path=w314) -> (string=w313:string)
        n138 = Concatenate Strings(w313, ".pdf" ("string")) -> (w311:string)
        n139 = String To Path(string=w311) -> (path=w275:path)
        n140 = call <vilib>:"Excel Get ActiveX References.vi"("report in"=w277, "error in (no error)"=w279) -> ("report out"=w276:refnum<class "NI_report.lvclass">, "Excel._Worksheet"=w284:refnum<k7>, "error out"=w281:errorcluster)  [unwired: 7 in, 4 out]
        n141 = invoke class="_Worksheet" method="ExportAsFixedFormat"(reference=w284, error in=w281, "Type"=w283, "Filename"=w275, "OpenAfterPublish"=TRUE) -> (error out=w278:errorcluster)  [unwired: 7 in, 11 out]
        n142 = call-dynamic "Dispose Report.vi"("report in"=w276, "error in (no error)"=w278) -> ("error out"=w315:errorcluster)  [unwired: 13 in]
        n143 = flat-sequence {
          tunnel: w315 -> [w343]
          tunnel: [w343] -> w316
          frame #0 {
            n144 = local write "Status bar"("Completed" ("Status bar")) -> ()
          }
        }
      }
    }
    n145 = call <vilib>:"Simple Error Handler.vi"("error in (no error)"=w66) -> ("error out"=w65:errorcluster)  [unwired: 4 in, 4 out]
    n146 = Wait (ms)(milliseconds to wait=u32 500) -> ()  [unwired: 1 out]
  }
  n147 = call <vilib>:"DB Tools Close Connection.vi"("error in (no error)"=w45, "connection reference"=w44) -> ("error out"=w2:errorcluster)  [unwired: 5 in]
  n148 = call <vilib>:"Clear Errors.vi"("error in (no error)"=w2) -> ("error out"=w1:errorcluster)  [unwired: 5 in, 1 out]
  n149 = flat-sequence {
    tunnel: [w352] -> w21
    tunnel: w1 -> [w353]
    frame #0 {
      n150 = property class="App"(error in=w353) -> (error out=w354:errorcluster, "App.Kind"=w355:T17)  [unwired: 1 in, 1 out]
      n151 = case shown="\"Run Time System\"" w355 {
        tunnel: w354 -> [w356 w358]
        tunnel: [w356 w357] -> w352
        frame Default {
        }
        frame "Run Time System" {
          n152 = invoke class="VI" method="FP.Close"(error in=w358) -> (error out=w357:errorcluster)  [unwired: 2 in, 2 out]
        }
      }
    }
  }
  "error out" <- w21
